vi "Get_Randomized_Image_Name-2.vi"(2 "error IN":errorcluster, 3 "[IN] Main Name":string) -> (0 "error OUT":errorcluster, 1 "[OUT] Randomized name":string)   [LabVIEW 2017]
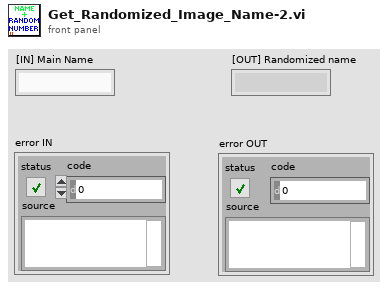
[diagram p1: front panel]
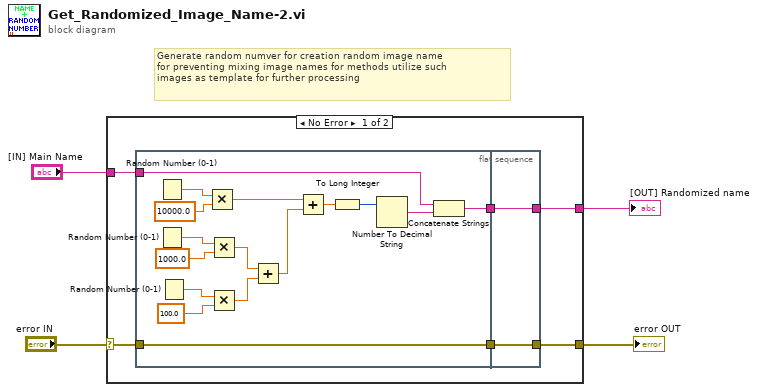
[diagram p0: block diagram]
diagram:
  # "Generate random numver for creation random image name \nfor preventing mixing image names for methods utilize such\nimages as template for further processing"
  n1 = case shown="No Error" "error IN" {
    selector: "error IN" -> [w7 w29]
    tunnel: "[IN] Main Name" -> [w10 w30]
    tunnel: [w9 w30] -> w3
    tunnel: [w5 w29] -> w1
    frame No Error {
      n2 = flat-sequence {
        tunnel: w10 -> [w26]
        tunnel: [w25] -> w8
        tunnel: w7 -> [w11]
        tunnel: [w11] -> w6
        tunnel: [w28] -> w9
        tunnel: w8 -> [w28]
        tunnel: [w27] -> w5
        tunnel: w6 -> [w27]
        frame #0 {
          n3 = Random Number (0-1)() -> (number: 0 to 1=w21:dbl)
          n4 = Random Number (0-1)() -> (number: 0 to 1=w20:dbl)
          n5 = Random Number (0-1)() -> (number: 0 to 1=w18:dbl)
          n6 = Multiply(x=w21, y=10000.0) -> (x*y=w14:dbl)
          n7 = Multiply(x=w20, y=1000.0) -> (x*y=w16:dbl)
          n8 = Multiply(x=w18, y=100.0) -> (x*y=w15:dbl)
          n9 = Add(x=w16, y=w15) -> (x+y=w13:dbl)
          n10 = Add(x=w14, y=w13) -> (x+y=w12:dbl)
          n11 = To Long Integer(number=w12) -> (32bit integer=w24:i32)
          n12 = Number To Decimal String(number=w24) -> (decimal integer string=w23:string)  [unwired: 1 in]
          n13 = Concatenate Strings(w26, w23) -> (w25:string)
        }
        frame #1 {
        }
      }
    }
    frame Error {
    }
  }
  "error OUT" <- w1
  "[OUT] Randomized name" <- w3
